vi "Blending Objects.vi"() -> ()   [LabVIEW 2016]
doc: "This VI shows how to use blending effects to create transparent objects. It also shows different operations with objects, like Culling Effects or Draw Styles."
uses:
  <vilib>/picture/3D Picture Control/Object/Create Object (drawable).vi
  <vilib>/picture/3D Picture Control/Object/Create Object (name).vi
  <vilib>/picture/3D Picture Control/Object/Add Object (no reference).vi
  <vilib>/picture/3D Picture Control/NI_3D Picture Control.lvlib
panel:
  in  "Alpha Box":dbl(slide)=0.3 scale=0.0..1.0
  in  "Box Length for Y-axis":sgl(slide)=7.7 scale=0.1..10.0
  in  "Box Draw Style":T1(ring)=enum."Polygons"
  in  "Ball Size":sgl(slide)=1.0 scale=1.0..5.0
  in  "Box Blending Mode":enum16{"Inherit Value", "Off", "On"}(ring)=enum."On"
  in  "Box Facing Culling":T2(ring)=enum."No Culling"
  in  "Stop":bool
  in  "Type of Blending (Bin)":T3(ring)=enum."Transparent Bin"
  out "3D Picture":refnum<vi>(3d-picture)
  # "Overview: This VI shows how to use blending effects to create transparent objects in a 3D Picture.\nRequirements: LabVIEW Full Development System\nInstructions: \n1. Run the VI.\n2. Change the Box Length for Y-axis and Ball Size to change the size of the box and the ball.\n3. Change the Box Facing Culling value and observe how it affects the box.\n4. Change the Type of Blending (Bin) to observe the other options available for rendering.\n5. Change the Box Blending Mode to see how the 3D Picture would render if you did not have blending.\n6. Click Stop to stop the VI."
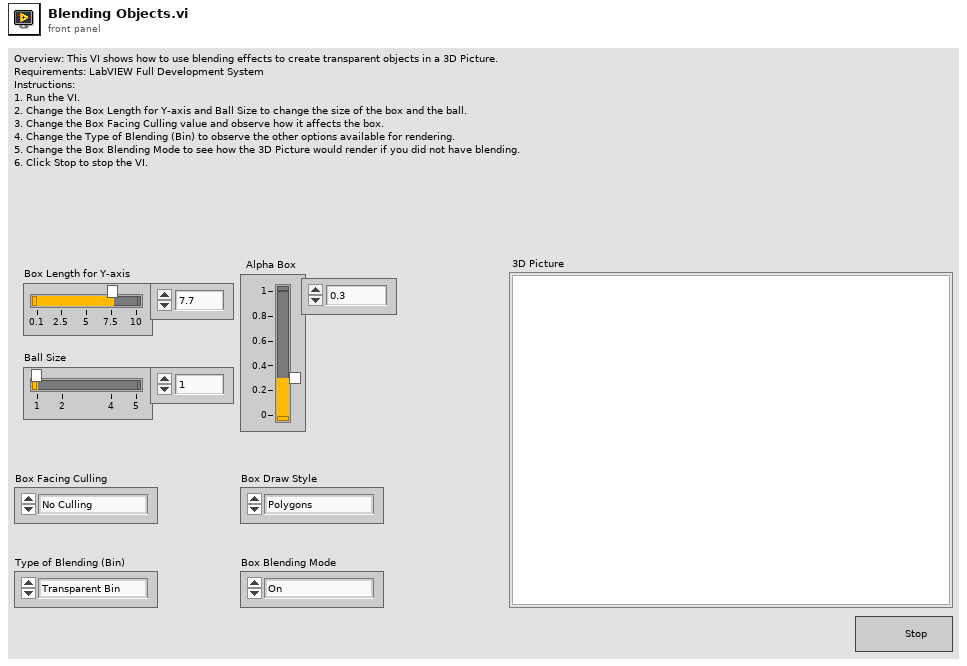
[diagram p1: front panel]
types:
  T1 = enum16{"Inherit Value", "Points", "Wireframe", "Polygons"}
  T2 = enum16{"Inherit Value", "No Culling", "Cull Back Face", "Cull Front Face", "Cull Both Faces"}
  T3 = enum16{"Normal Bin", "Opaque Bin", "Transparent Bin"}
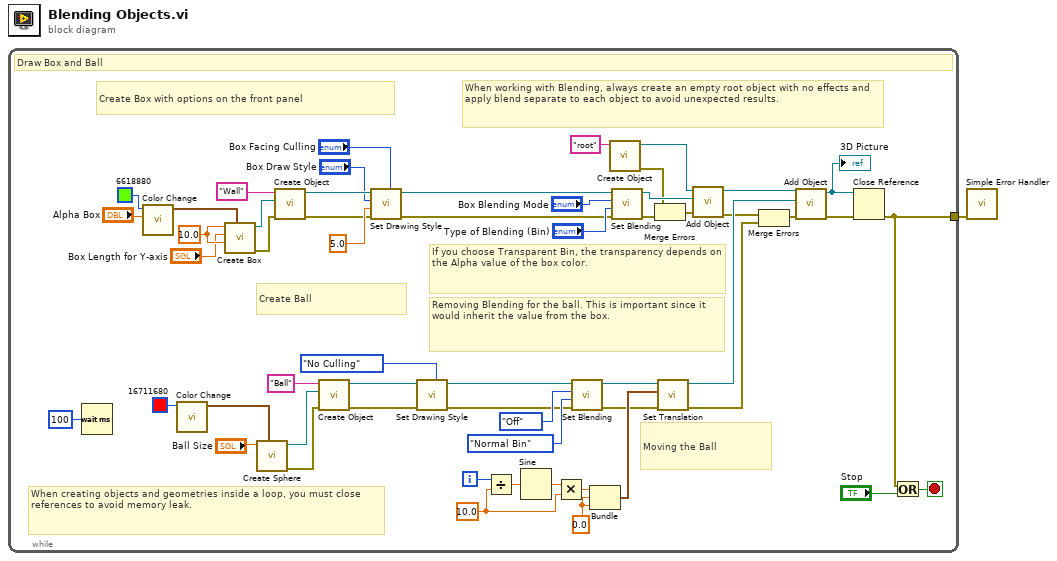
[diagram p0: block diagram]
diagram:
  n1 = while {
    tunnel: [w2] -> w1
    i -> [w40]
    stop <- w16 stop-if-true
    w32 = sgl 10.0 ("Length Z")
    w33 = 10.0 ("x")
    w38 = 0.0 ("sin(x)")
    # "When creating objects and geometries inside a loop, you must close references to avoid memory leak."
    # "If you choose Transparent Bin, the transparency depends on the Alpha value of the box color."
    # "When working with Blending, always create an empty root object with no effects and apply blend separate to each object to avoid unexpected results."
    # "Create Ball"
    # "Create Box with options on the front panel"
    # "Moving the Ball"
    # "Removing Blending for the ball. This is important since it would inherit the value from the box."
    # "Draw Box and Ball"
    n2 = Wait (ms)(milliseconds to wait=u32 100 ("millisecond multiple")) -> ()  [unwired: 1 out]
    n3 = call <vilib>:"Color Change.vi"("Alpha"="Alpha Box", "Color"=u32 6618880) -> ("RGBA"=w45:cluster{"R":sgl, "G":sgl, "B":sgl, "A":sgl})  [unwired: 9 in]
    n4 = call <vilib>:"Color Change.vi"("Color"=u32 16711680) -> ("RGBA"=w48:cluster{"R":sgl, "G":sgl, "B":sgl, "A":sgl})  [unwired: 10 in]
    n5 = call <vilib>:"Create Box.vi"("Color"=w45, "Length Z"=w32, "Length Y"="Box Length for Y-axis", "Length X"=w32) -> ("error out"=w26:errorcluster, "New Box Refnum"=w51:refnum<vi>)  [unwired: 6 in]
    n6 = call <vilib>:"Create Sphere.vi"("Color"=w48, "Radius"="Ball Size") -> ("error out"=w30:errorcluster, "New Sphere Refnum"=w49:refnum<vi>)  [unwired: 8 in]
    n7 = call-poly <vilib>:"Create Object.vi"("error in (no error)"=w26, "Geometry"=w51, "Name"="Wall") -> ("error out"=w5:errorcluster, "Scene:New Object"=w25:refnum<vi>)  [unwired: 7 in]
    n8 = call-poly <vilib>:"Create Object.vi"("error in (no error)"=w30, "Geometry"=w49, "Name"="Ball") -> ("error out"=w6:errorcluster, "Scene:New Object"=w20:refnum<vi>)  [unwired: 7 in]
    n9 = call <vilib>:"Set Drawing Style.vi"("Face Culling Mode"="Box Facing Culling", "error in (no error)"=w5, "Size"=5.0, "Mode"="Box Draw Style", "Scene Object In"=w25) -> ("error out"=w22:errorcluster, "Scene Object Out"=w23:refnum<vi>)  [unwired: 5 in]
    n10 = call <vilib>:"Set Drawing Style.vi"("Face Culling Mode"=T2."No Culling" ("Draw Style:Face Culling Mode"), "error in (no error)"=w6, "Scene Object In"=w20) -> ("error out"=w17:errorcluster, "Scene Object Out"=w18:refnum<vi>)  [unwired: 7 in]
    n11 = Divide(x=w40, y=w33) -> (x/y=w34:dbl)
    n12 = Sine(x=w34) -> (sin(x)=w39:dbl)
    n13 = Multiply(x=w39, y=w33) -> (x*y=w35:dbl)
    n14 = call <vilib>:"Set Blending.vi"("error in (no error)"=w17, "Bin"=T3."Normal Bin" ("Blending:Bin"), "Mode"=enum16{"Inherit Value", "Off", "On"}."Off" ("Specials:Depth Test"), "Scene Object In"=w18) -> ("error out"=w29:errorcluster, "Scene Object Out"=w42:refnum<vi>)  [unwired: 6 in]
    n15 = Bundle(w35, "sin(x)"=w38, "sin(x)"=w38) -> (w37:cluster{dbl, "sin(x)":dbl, "sin(x)":dbl})  [unwired: 1 in]
    n16 = call-poly <vilib>:"Create Object.vi"("Name"="root") -> ("error out"=w9:errorcluster, "Scene:New Object"=w13:refnum<vi>)  [unwired: 9 in]
    n17 = call <vilib>:"Set Blending.vi"("error in (no error)"=w22, "Bin"="Type of Blending (Bin)", "Mode"="Box Blending Mode", "Scene Object In"=w23) -> ("error out"=w8:errorcluster, "Scene Object Out"=w14:refnum<vi>)  [unwired: 6 in]
    n18 = Merge Errors(w9, w8) -> (w7:errorcluster)
    n19 = call <vilib>:"Set Translation.vi"("error in (no error)"=w29, "Translation"=w37, "Scene Object"=w42) -> ("error out"=w28:errorcluster, "Translated Object"=w41:refnum<vi>)  [unwired: 7 in]
    n20 = call-poly <vilib>:"Add Object.vi"("error in (no error)"=w7, "New Object In"=w14, "Scene Object In"=w13) -> ("error out"=w10:errorcluster, "Scene Object Out"=w12:refnum<vi>)  [unwired: 7 in]
    n21 = Merge Errors(w10, w28) -> (w27:errorcluster)
    n22 = call-poly <vilib>:"Add Object.vi"("error in (no error)"=w27, "New Object In"=w41, "Scene Object In"=w12) -> ("error out"=w4:errorcluster, "Scene Object Out"=w3:refnum<vi>)  [unwired: 7 in]
    "3D Picture" <- w3
    n23 = Close Reference(reference=w3, error in (no error)=w4) -> (error out=w2:errorcluster)
    n24 = Or(x=w2, y="Stop") -> (x .or. y?=w16:bool)
  }
  n25 = call <vilib>:"Simple Error Handler.vi"("error in (no error)"=w1) -> ()  [unwired: 4 in, 5 out]
